vi "Write Block Color.vi"(8 "error in (no error)":errorcluster, 10 "Block Color":u32(colorbox), 11 "XYGraphOverview in":refnum<class "XYGraphOverview.lvclass">) -> (0 "error out":errorcluster, 3 "XYGraphOverview out":refnum<class "XYGraphOverview.lvclass">)   [LabVIEW 2020, in "XYGraphOverview.lvlib" / "XYGraphOverview.lvclass"]
uses:
  XYGraphOverview.lvclass
  XYGraphOverview.lvclass/XYGraphOverview.ctl
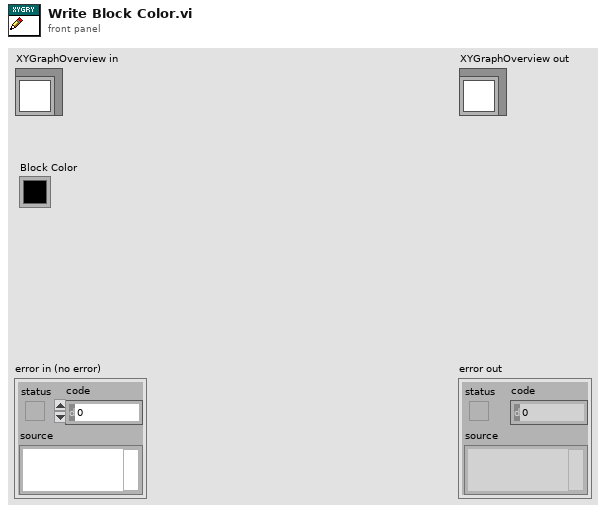
[diagram p1: front panel]
types:
  T1 = typedef "XYGraphOverview.lvlib/XYGraphOverview.lvclass/State Data.ctl" = cluster{"Sample Multiplier":u32, "Block Color":u32, "Highlight Color":u32}
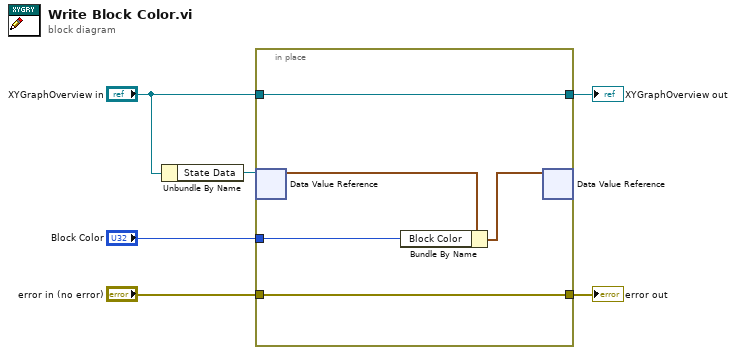
[diagram p0: block diagram]
diagram:
  n1 = Unbundle By Name("XYGraphOverview in") -> ("State Data"=w6:refnum<data-value>)
  n2 = in-place {
    in-place-border: "XYGraphOverview in" -> [w11]
    in-place-border: [w11] -> w2
    in-place-border: "error in (no error)" -> [w10]
    in-place-border: [w10] -> w3
    in-place-border: "Block Color" -> [w7]
    n3 = in-place-dvr #1(w6) -> (w9:T1)  [unwired: 1 out]
    n4 = Bundle By Name(cluster=w9, "Block Color"=w7) -> (w8:T1)
    n5 = in-place-dvr #1(w8) -> ()  [unwired: 2 out]
  }
  "error out" <- w3
  "XYGraphOverview out" <- w2
